vi "查找空元素.vi"(6 "error in (no error)":errorcluster caption="错误输入（无错误）", 8 "offset (0)":i32 caption="偏移量(0)", 11 "XML String In":string caption="XML字符串输入") -> (0 "offset past match":i32 caption="匹配后偏移量", 1 "after  tag":string caption="标识符之后", 2 "tag":string caption="标识符", 3 "before tag":string caption="标识符之前", 4 "error out":errorcluster caption="错误输出", 5 "element name":string caption="元素名", 7 "node name":string caption="节点名")   [LabVIEW 2017]
uses:
  <vilib>/regexp/Match Regular Expression.xnode
panel:
  # "<编号 id=\"001\"/>"
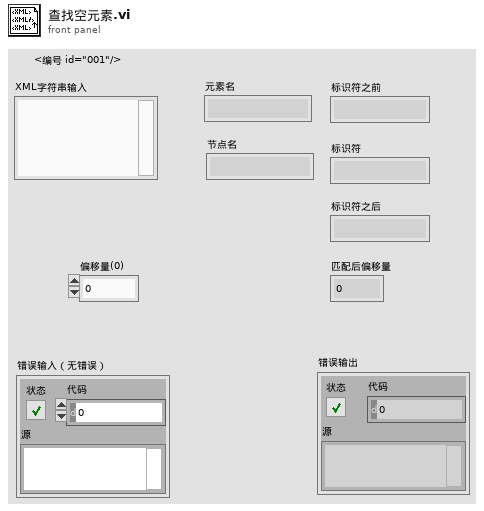
[diagram p1: front panel]
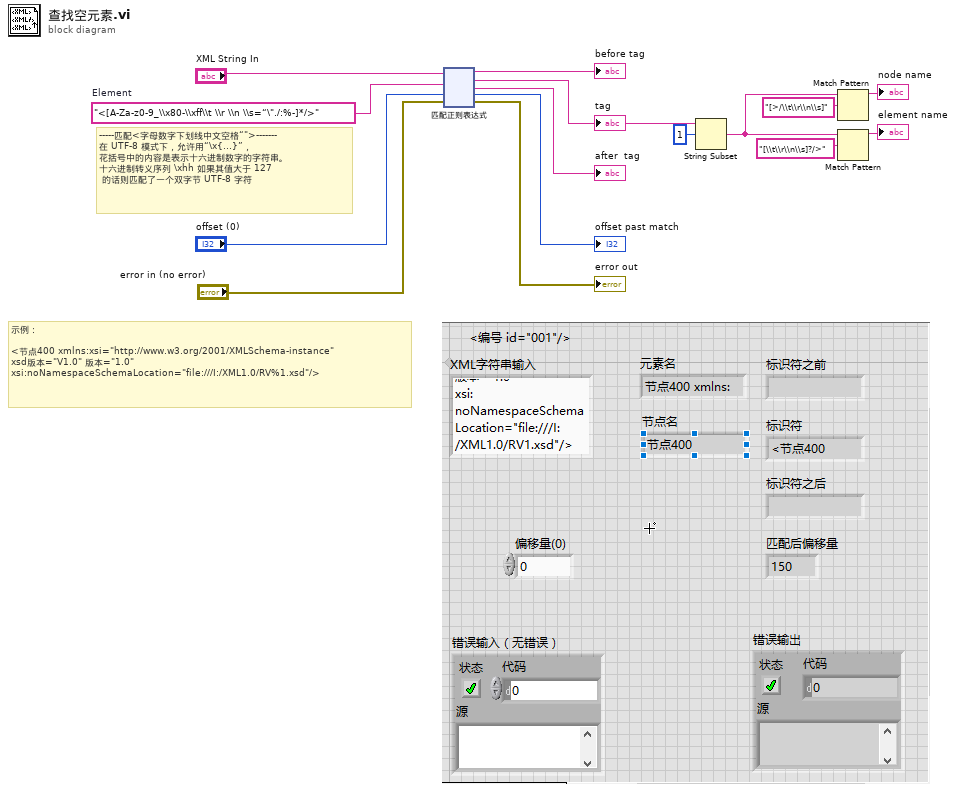
[diagram p0: block diagram]
diagram:
  w8 = "<[A-Za-z0-9_\\x80-\\xff\\t \\r \\n \\s=“\"./:%-]*/>"  # Element
  # "示例：\n\n<节点400 xmlns:xsi=\"http://www.w3.org/2001/XMLSchema-instance\" \nxsd版本=\"V1.0\" 版本=\"1.0\" \nxsi:noNamespaceSchemaLocation=\"file:///I:/XML1.0/RV%1.xsd\"/>"
  # "-----匹配<字母数字下划线中文空格“\">-------\n在 UTF-8 模式下，允许用“\\x{...}”，\n花括号中的内容是表示十六进制数字的字符串。\n十六进制转义序列 \\xhh 如果其值大于 127\n 的话则匹配了一个双字节 UTF-8 字符"
  n1 = xnode "匹配正则表达式"("输入字符串"="XML String In", "正则表达式"=w8, "偏移量(0)"="offset (0)", "错误输入"="error in (no error)") -> ("匹配之前"=→"before tag":string, "所有匹配"=w10:string, "匹配之后"=→"after  tag":string, "匹配后偏移量"=→"offset past match":i32, "错误输出"=→"error out":errorcluster)  [unwired: 2 in]
  "tag" <- w10
  n2 = String Subset(string=w10, offset (0)=1) -> (substring=w1:string)  [unwired: 1 in]
  n3 = Match Pattern(string=w1, regular expression="[>/\\t\\r\\n\\s]") -> (before substring=→"node name":string)  [unwired: 1 in, 3 out]
  n4 = Match Pattern(string=w1, regular expression="[\\t\\r\\n\\s]?/>") -> (before substring=→"element name":string)  [unwired: 1 in, 3 out]
